vi "basis_(subvi).vi"() -> ()   [LabVIEW 2015]
panel:
  in  "c":dbl
  in  "y1":dbl
  in  "y0":dbl
  in  "d":dbl
  out "phases":dbl[](array[numeric])
  out "coeffs":dbl[](array[numeric])
  out "modes":dbl[](array[numeric])
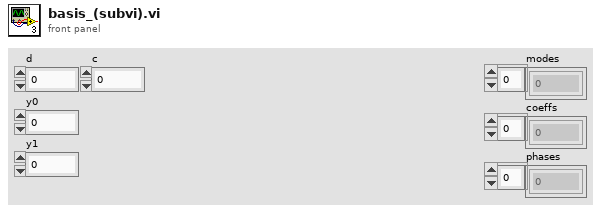
[diagram p1: front panel]
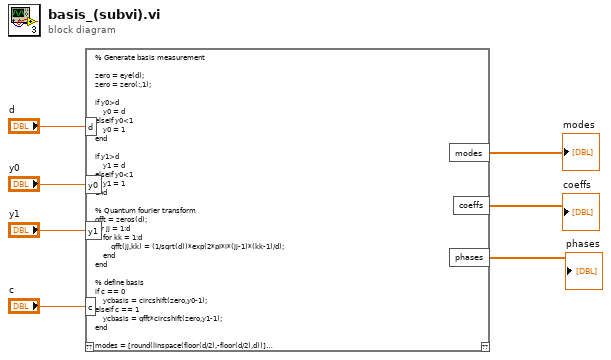
[diagram p0: block diagram]
diagram:
  n1 = script code="% Generate basis measurement\n\nzero = eye(d);\nzero = zero(:,1);\n\nif y0>d \n    y0 = d\nelseif y0<1\n    y0 = 1\nend\n\nif y1>d \n    y1 = d\nelseif y0<1\n    y1 = 1\nend\n\n% Quantum fourier transform\nqfft = zeros(d);\nfor jj = 1:d\n    for kk = 1:d\n        qfft(jj,kk) = (1/sqrt(d))*exp(2*pi*i*(jj-1)*(kk-1)/d);\n    end\nend\n\n% define basis\nif c == 0\n    ycbasis = circshift(zero,y0-1);\nelseif c == 1\n    ycbasis = qfft*circshift(zero,y1-1);\nend\n\nmodes = [round(linspace(floor(d/2),-floor(d/2),d))]\ncoeffs = [abs(ycbasis)]'\nphases = [angle(ycbasis)]'"("d"="d", "c"="c", "y0"="y0", "y1"="y1") -> ("modes"=→"modes":dbl[], "coeffs"=→"coeffs":dbl[], "phases"=→"phases":dbl[])  [unwired: 1 in, 1 out]
